vi "GetSwerveRawAzimuth.vi"(1 "Calibrate Wheels":bool, 2 "Azimuth Falcon Refnum":string="My Motor RefNum") -> (0 "Position (Raw Sensor Units)":i32)   [LabVIEW 2020]
doc: "Gets the raw azimuth position from the non-absolute encoder on the Falcon. Handles motor controller and RoboRIO brownout scenarios. Re-zeroing the swerve modules also occurs here."
uses:
  GRNF_CTREMotor.vi
  <vilib>/Rock Robotics/WPI/ThirdParty/Phoenix-LabVIEW/Motor Controller/Get/CTRE_Phoenix_MotorController_GetGeneralStatus.vi
  <vilib>/Rock Robotics/WPI/ThirdParty/Phoenix-LabVIEW/Motor Controller/Get/CTRE_Phoenix_MotorController_GetSelectedSensorData.vi
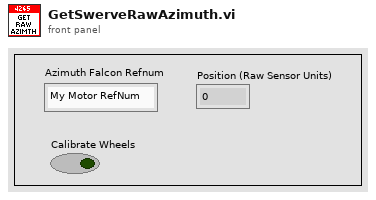
[diagram p1: front panel]
types:
  T1 = typedef "WPI_MotorControlDeviceRef.ctl" = cluster{"DeviceStatus":errorcluster, "Type":T2, "PWM":cluster{"PWM Channel":T3, "DeadBand":T4}, "CAN":cluster{"Device Number":u8, "SetOutput VI Ref":variant, "GetOutput VI Ref":variant, "Enable VI Ref":variant, "Disable VI Ref":variant, "Data":variant}, "Invert":bool, "DIO PWM":cluster{"PWM \"Enable\" Channel":T3, "DIOChannel":T5, "PWM Rate":dbl}}
  T2 = typedef "WPI_MotorControlType.ctl" = enum16{"PWM", "CAN", "DIO PWM"}
  T3 = typedef "FPGA_DIOPWMChannel.ctl" = enum8{"PWM 0", "PWM 1", "PWM 2", "PWM 3", "PWM 4", "PWM 5", "PWM 6", "PWM 7", "PWM 8", "PWM 9", "PWM MXP 0", "PWM MXP 1", "PWM MXP 2", "PWM MXP 3", "PWM MXP 4", "PWM MXP 5", "PWM MXP 6", "PWM MXP 7", "PWM MXP 8", "PWM MXP 9", "Invalid"}
  T4 = typedef "WPI_PWMDeadband.ctl" = cluster{"Name":string, "maxPositivePwm":i32, "minPositivePwm":i32, "centerPwm":i32, "maxNegativePwm":i32, "minNegativePwm":i32, "angularRange":u16}
  T5 = typedef "FPGA_DIOChannel.ctl" = enum8{"DIO 0", "DIO 1", "DIO 2", "DIO 3", "DIO 4", "DIO 5", "DIO 6", "DIO 7", "DIO 8", "DIO 9", "DIO MXP 0", "DIO MXP 1", "DIO MXP 2", "DIO MXP 3", "DIO MXP 4", "DIO MXP 5", "DIO MXP 6", "DIO MXP 7", "DIO MXP 8", "DIO MXP 9", "DIO MXP 10", "DIO MXP 11", "DIO MXP 12", "DIO MXP 13", "DIO MXP 14", "DIO MXP 15", "SPI Port CS1", "SPI Port CS2", "SPI Port CS3", "SPI Port MISO", "SPI Port MOSI", "Invalid"}
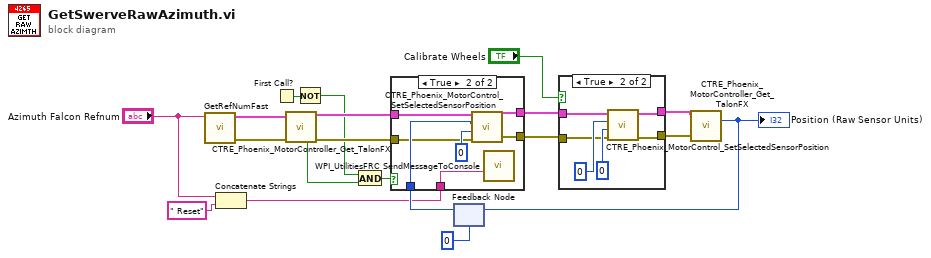
[diagram p0: block diagram]
diagram:
  n1 = call-poly "GetRefNumFast.vi"("RefNum Name"="Azimuth Falcon Refnum") -> ("Error"=w13:errorcluster, "Device Reference"=w12:T1)  [unwired: 5 in]
  n2 = Concatenate Strings("Azimuth Falcon Refnum", " Reset" ("string")) -> (w1:string)
  n3 = First Call?() -> (First Call?: T/F=w10:bool)
  n4 = call-poly <vilib>:"CTRE_Phoenix_MotorController_Get_TalonFX.vi"("PhoenixMotorControlDevRef"=w12, "error in"=w13) -> ("PhoenixMotorControlDevRef"=w14:T1, "Has Reset Occurred?"=w16:bool, "error out"=w15:errorcluster)  [unwired: 8 in, 3 out]
  n5 = Not(x=w10) -> (.not. x?=w11:bool)
  n6 = And(x=w11, y=w16) -> (x .and. y?=w9:bool)
  n7 = feedback #1(0 ("Position (Raw Sensor Units)")) -> (w6:i32)
  n8 = case shown="True" w9 {
    tunnel: w15 -> [w20 w25]
    tunnel: w14 -> [w21 w28]
    tunnel: [w21 w24] -> w7
    tunnel: [w20 w23] -> w8
    tunnel: w6 -> [_ w27]
    tunnel: w1 -> [_ w22]
    frame False {
    }
    frame True {
      n9 = call <vilib>:"CTRE_Phoenix_MotorControl_SetSelectedSensorPosition.vi"("error in (no error)"=w25, "pidLoopIdx"=u32 0, "New Sensor Position"=w27, "PhoenixMotorControlDevRef"=w28) -> ("error out"=w23:errorcluster, "PhoenixMotorControlDevRef"=w24:T1)  [unwired: 6 in]
      n10 = call <vilib>:"WPI_UtilitiesFRC SendMessageToConsole.vi"("Message"=w22) -> ()  [unwired: 14 in, 1 out]
    }
  }
  n11 = case shown="True" "Calibrate Wheels" {
    tunnel: w8 -> [w29 w31]
    tunnel: w7 -> [w30 w34]
    tunnel: [w30 w35] -> w17
    tunnel: [w29 w36] -> w18
    frame False {
    }
    frame True {
      n12 = call <vilib>:"CTRE_Phoenix_MotorControl_SetSelectedSensorPosition.vi"("error in (no error)"=w31, "pidLoopIdx"=u32 0, "New Sensor Position"=0, "PhoenixMotorControlDevRef"=w34) -> ("error out"=w36:errorcluster, "PhoenixMotorControlDevRef"=w35:T1)  [unwired: 6 in]
    }
  }
  n13 = call-poly <vilib>:"CTRE_Phoenix_MotorController_Get_TalonFX.vi"("PhoenixMotorControlDevRef"=w17, "error in"=w18) -> ("Position (Raw Sensor Units)"=w19:i32)  [unwired: 10 in, 3 out]
  "Position (Raw Sensor Units)" <- w19
  n14 = feedback-in #1(w19) -> ()
